vi "Cal Inst - raw to waveform array.vi"(7 "String":string, 8 "error in (no error)":errorcluster, 9 "seconds since 1Jan1904":timestamp, 10 "Numeric":dbl, 11 "output string":string) -> (0 "error out":errorcluster, 3 "Waveform":waveform(sgl))   [LabVIEW 2013, in "Cal Inst Acquisition.lvlib"]
uses:
  Cal Inst Acquisition.lvlib
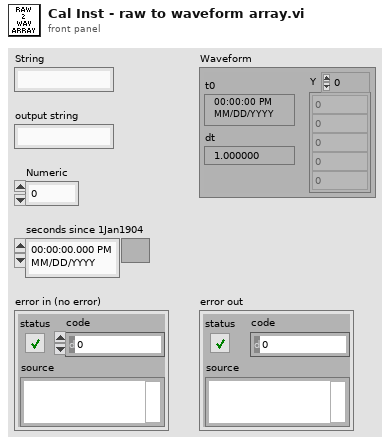
[diagram p1: front panel]
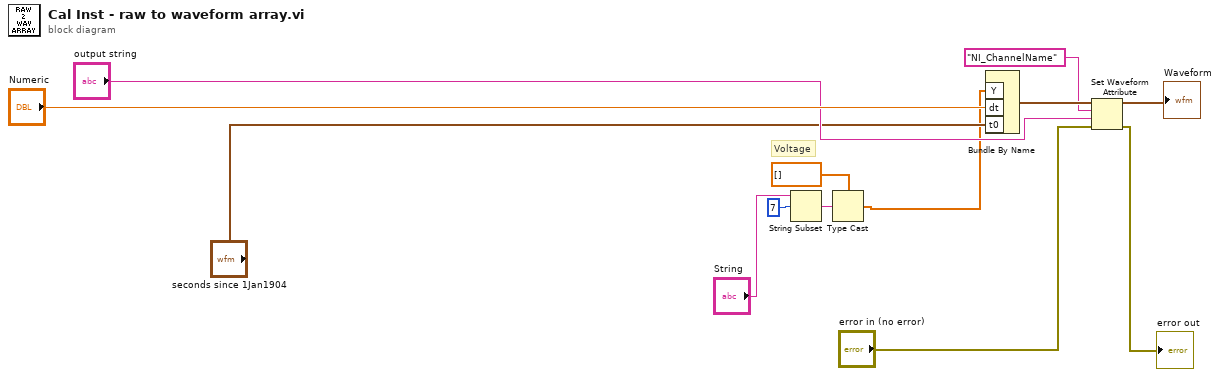
[diagram p0: block diagram]
diagram:
  # "Voltage"
  n1 = String Subset(string="String", offset (0)=7) -> (substring=w2:string)  [unwired: 1 in]
  n2 = Type Cast(type=sgl[] [], x=w2) -> (*(type *) &x=w7:sgl[])
  n3 = Bundle By Name("Y"=w7, "dt"="Numeric", "t0"="seconds since 1Jan1904") -> (w6:waveform(sgl))  [unwired: 1 in]
  n4 = Set Waveform Attribute(4:"error in (no error)", 5:"output string", 6:"NI_ChannelName" ("name"), 7:w6) -> (0:→"error out":errorcluster, 3:→"Waveform":waveform(sgl))  [unwired: 1 out]
